vi "一体站流程自动启动.vi"(11 "参数":T1={"CODCr"={"启动测量模式"={"测量模式"=enum."水样测量"}, "确定按钮"=TRUE}, "参数启用"={"多参数"=FALSE, "CODMn"=FALSE, "总磷总氮"=FALSE, "氨氮"=FALSE, "CODcr"=FALSE}}) -> ()   [LabVIEW 2016, in "PLC.lvlib"]
uses:
  PLC.lvlib
  API/CodCr/CodCr.lvlib
panel:
  out "枚举":enum16{"初始化", "采配水启动", "等待", "配水", "排水", "结束"}(ring)
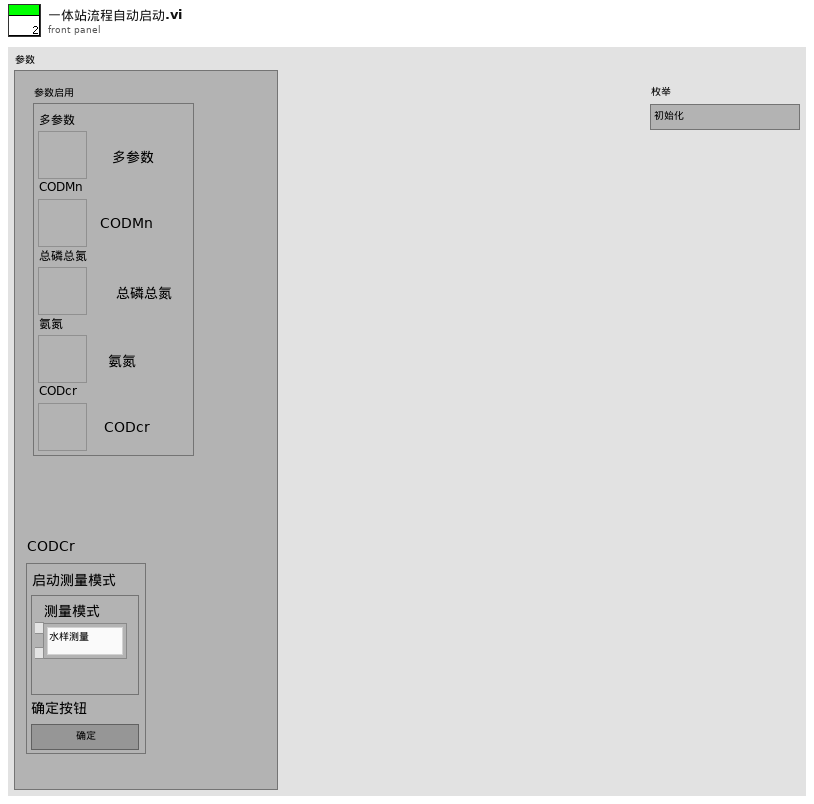
[diagram p1: front panel]
types:
  T1 = cluster{"CODCr":cluster{"启动测量模式":cluster{"测量模式":enum16{"水样测量", "标样核查", "零点核查", "加标回收", "平行样", "校零", "校标"}}, "确定按钮":bool}, "参数启用":cluster{"多参数":bool, "CODMn":bool, "总磷总氮":bool, "氨氮":bool, "CODcr":bool}}
  T2 = cluster{"命令":string, cluster{"starting address":u16, "holding register value":u16}}
  T3 = enum16{"待机", "启动氨氮", "氨氮测量中", "启动总磷", "总磷测量中", "结束"}
  T4 = cluster{"站号":u16, "量程切换":enum32{"H", "L", "AUTO"}, "控制命令":enum16{"启动测量", "标样核查", "零点核查", "跨度核查", "空白测试", "平行样测试", "加标回收", "空白校准", "标样校准", "初始化（清洗）", "停止测试", "仪器重启", "校时", "模式设置", "测量间隔设置"}, "模式设置":enum16{"待机", "连续模式", "周期模式", "定点模式", "受控模式", "手动模式"}, "测量间隔":u16}
  T5 = cluster{"时间标识":timestamp, "设备":string, "日志信息":string}
  T6 = cluster{"站号":u16, "量程切换":enum32{"H", "L", "AUTO"}, "控制命令":enum16{"启动测量", "标样核查", "零点核查", "跨度核查", "空白测试", "平行样测试", "加标回收", "空白校准", "标样校准", "初始化（清洗）", "停止测试", "仪器重启", "校时", "模式设置", "测量间隔设置", "盲样测试"}, "模式设置":enum16{"待机", "连续模式", "周期模式", "定点模式", "受控模式", "手动模式"}, "测量间隔":u16}
  T7 = enum16{"空闲", "水样测试", "标样核查", "零点核查", "跨度核查", "空白测试", "平行样测试", "加标回收", "空白校准", "标样校准", "初始化（清洗）"}
  T8 = cluster{"测量模式":enum16{"待机", "水样测试", "标样核查", "零点核查", "跨度核查", "空白测试", "平行样测试", "加标回收", "空白校准", "标样校准", "初始化（清洗）"}, "数据标记表":string, "测量时间":dbl}
  T9 = enum16{"待机", "水样测试", "标样核查", "零点核查", "跨度核查", "空白测试", "平行样测试", "加标回收", "空白校准", "标样校准", "初始化（清洗）"}
  T10 = cluster{"R0":i16, "R1":i16, "R2":i16, "R3":i16, "R4":i16, "R5":i16, "R6":i16, "R7":i16, "R8":i16, "R9":i16, "R10":i16, "R11":i16, "R12":i16, "R13":i16, "R14":i16, "R15":i16, "R16":i16, "R17":i16, "R18":i16, "R19":i16, "R20":i16, "R21":i16, "R22":i16}
  T11 = enum32{"Bad", "Idle", "Run top level", "Running"}
  T12 = cluster{"测量模式":enum16{"水样测量", "标样核查", "零点核查", "加标回收", "平行样", "校零", "校标"}}
  T13 = cluster{"系统时间":timestamp, "工作状态":enum16{"空闲", "水样测试", "标样核查", "零点核查", "跨度核查", "空白测试", "平行样测试", "加标回收", "空白校准", "标样校准", "初始化（清洗）"}, "测量模式":enum16{"待机", "连续模式", "周期模式", "定点模式", "受控模式", "手动模式"}, "告警代码":enum16{"无告警", "缺试剂告警", "缺水样告警", "缺蒸馏水告警", "缺标液告警", "仪表漏液告警", "标定异常告警", "超量程告警", "加热异常", "低试剂预警", "超上限告警", "超下限告警", "仪表内部其他异常", "滴定异常告警", "电极异常告警", "量程切换告警", "参数设置告警", "PH电极电位异常", "电导率电极异常", "浊度光度异常", "溶解氧电极异常", "溶解氧光强异常", "温度异常告警", "PH异常告警", "溶解氧异常告警", "电导率异常告警", "浊度异常告警", "叶绿素异常告警", "藻密度异常告警", "蓝绿藻异常告警", "ORP异常告警", "氨氮异常告警", "清洁刷异常告警", "SD卡异常告警", "蓝牙异常告警", "Wifi异常告警", "流程异常告警"}, "故障代码":enum16{"无故障", "电机故障", "温度故障", "通讯故障", "滴定故障"}, "日志代码":u16, "软件版本":u16, "F0":sgl, "F1":sgl, "F2":sgl, "F3":sgl, "T":sgl, "H":sgl, "id":u16, "flowid":u16, "量程":u16}
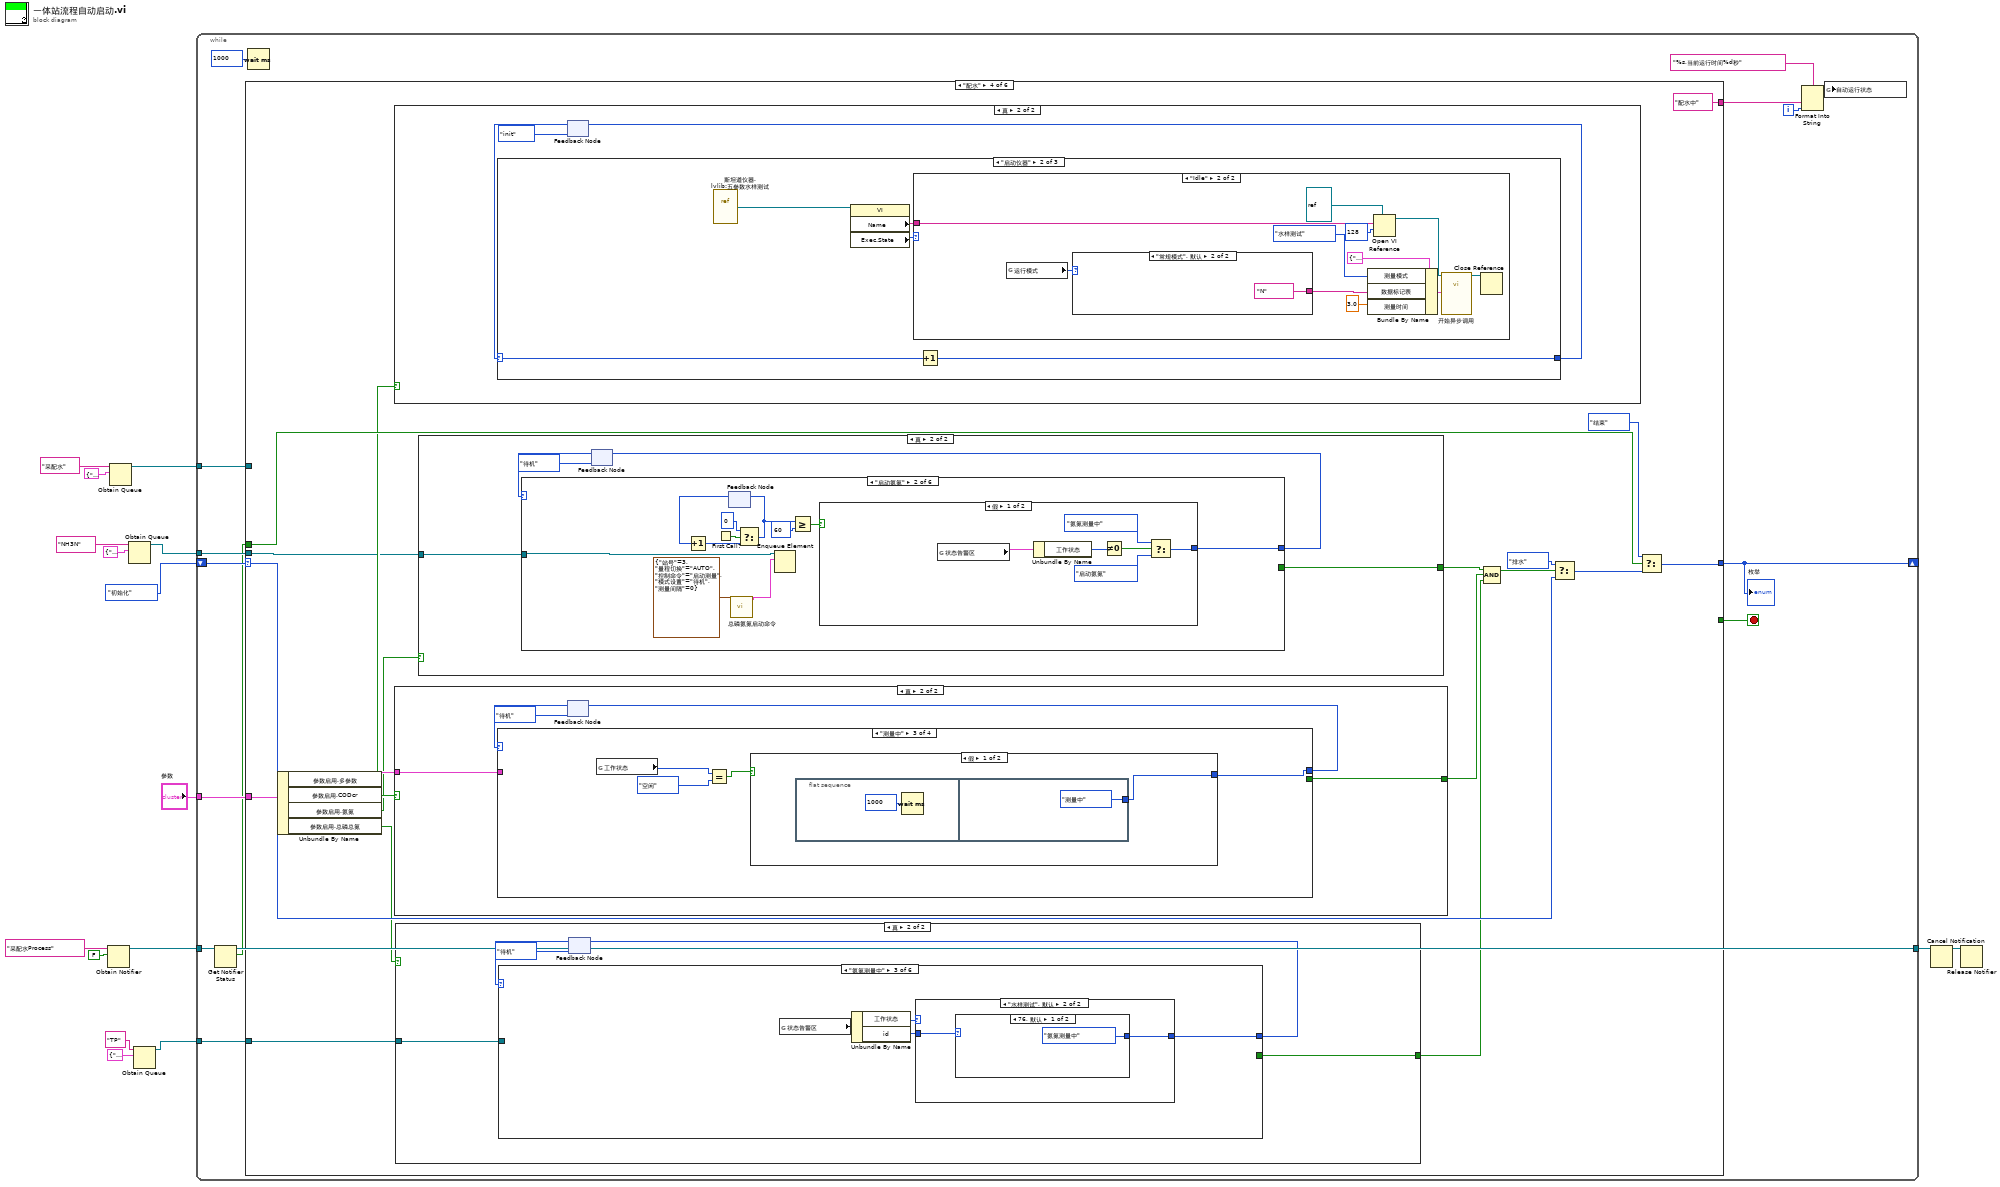
[diagram p0: block diagram]
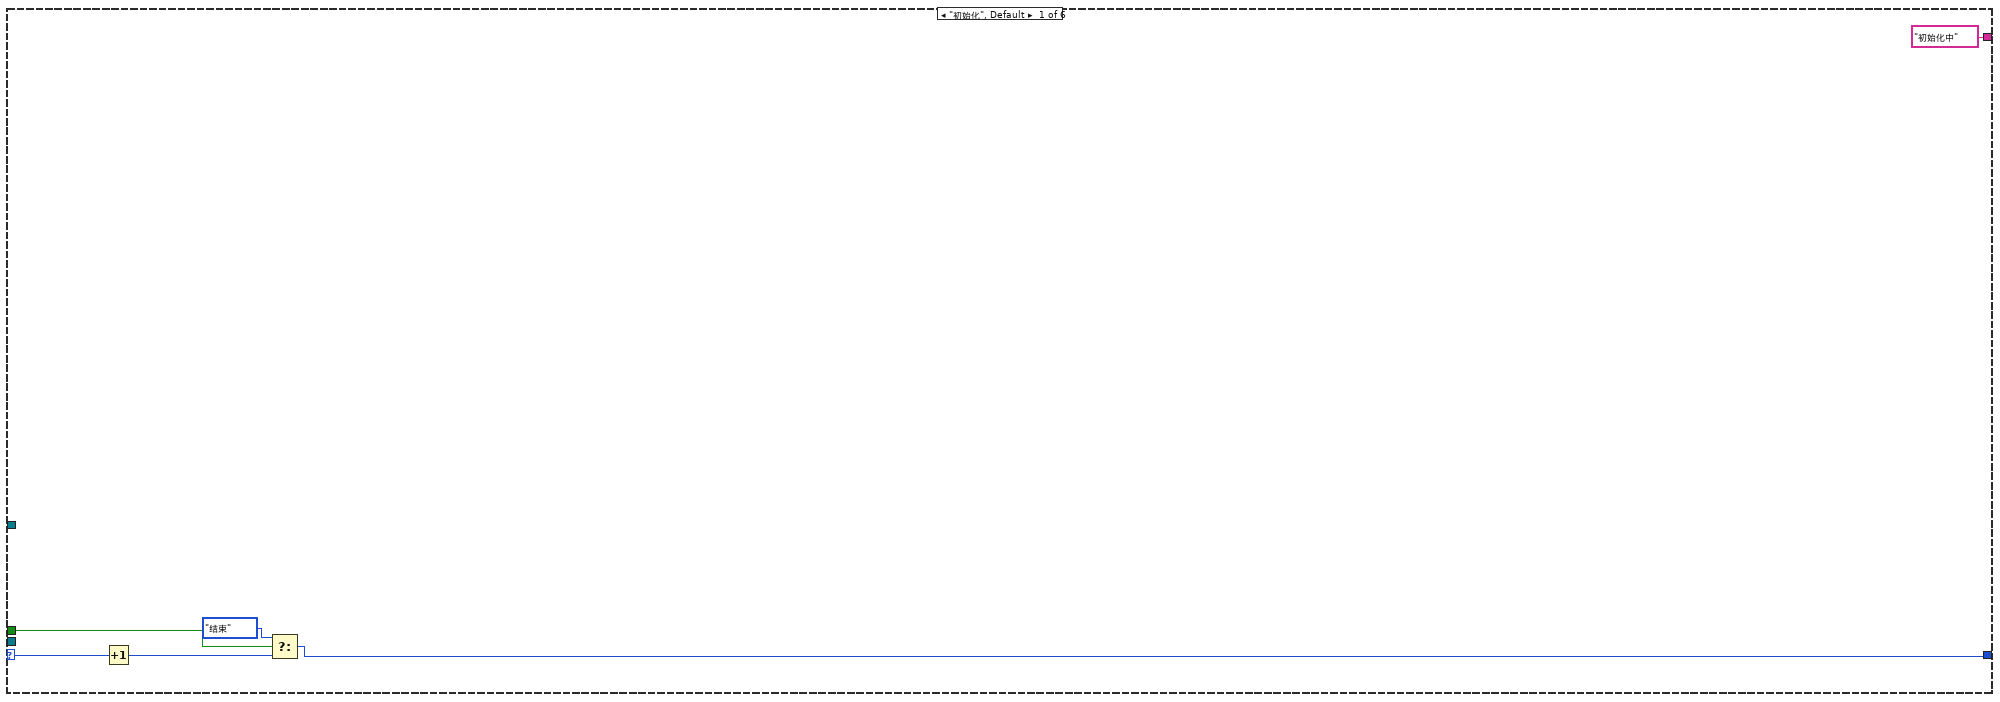
[diagram p2: hidden frame]
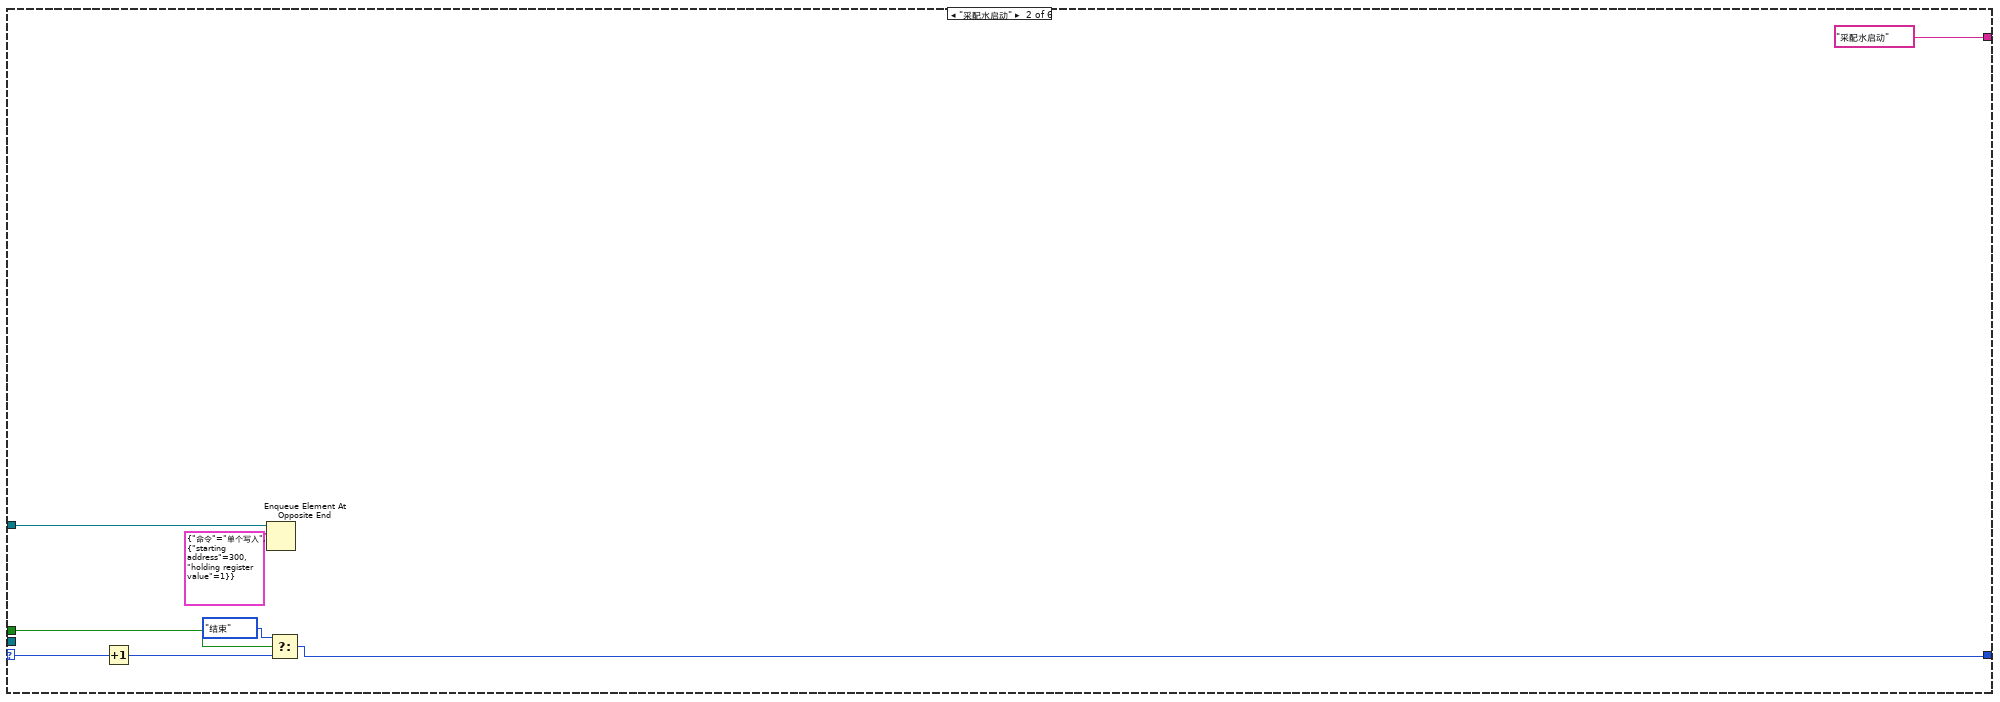
[diagram p3: hidden frame]
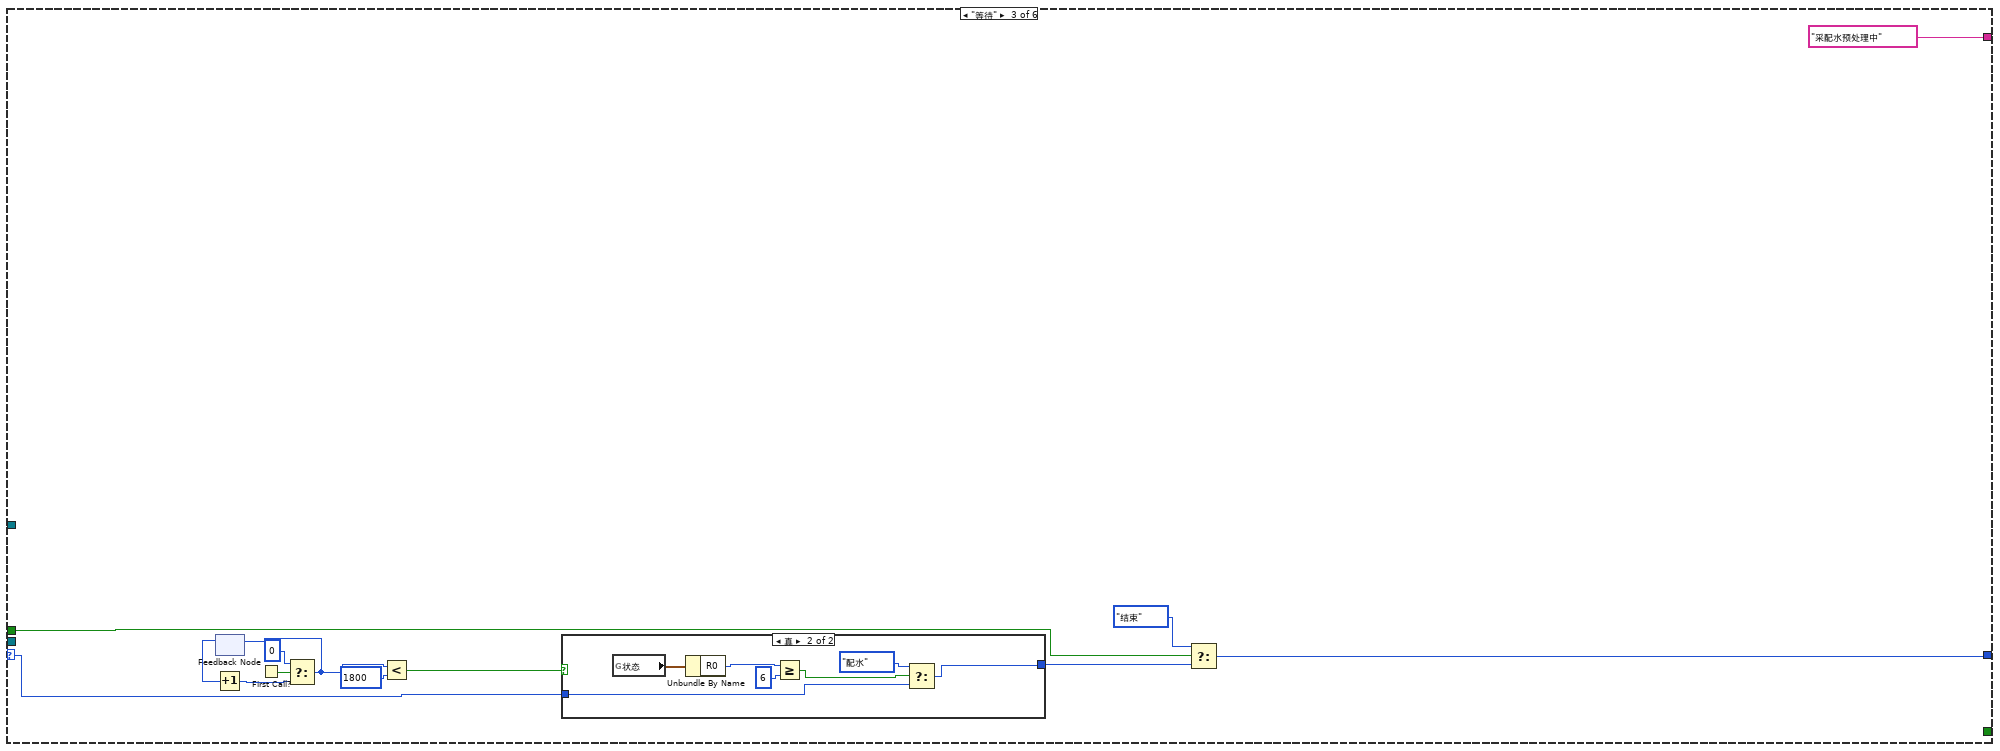
[diagram p4: hidden frame]
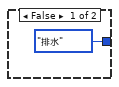
[diagram p5: hidden frame]
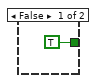
[diagram p6: hidden frame]
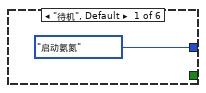
[diagram p7: hidden frame]
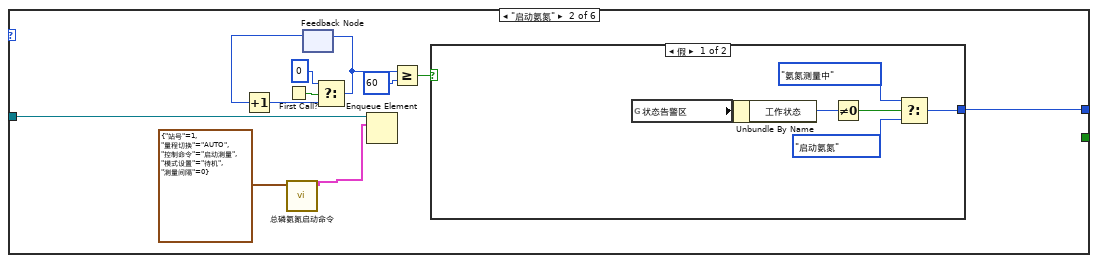
[diagram p8: hidden frame]
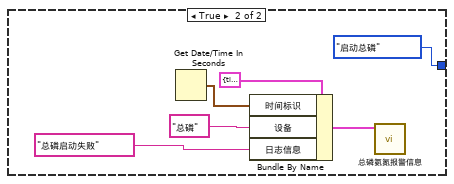
[diagram p9: hidden frame]
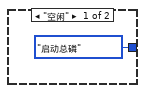
[diagram p10: hidden frame]
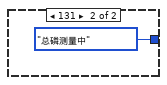
[diagram p11: hidden frame]
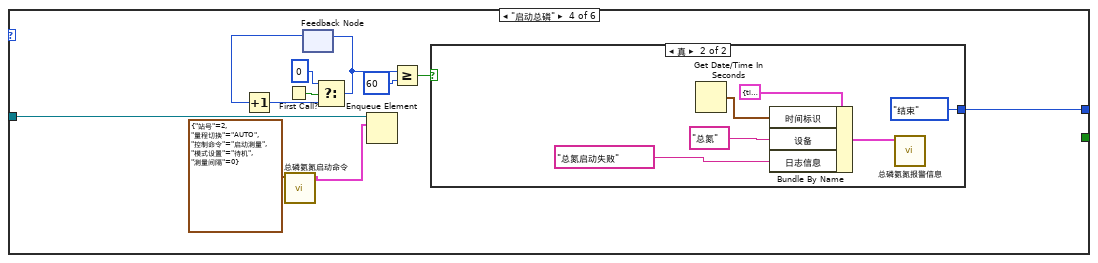
[diagram p12: hidden frame]
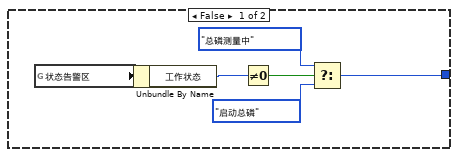
[diagram p13: hidden frame]
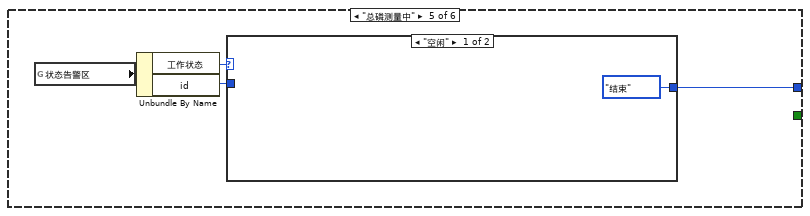
[diagram p14: hidden frame]
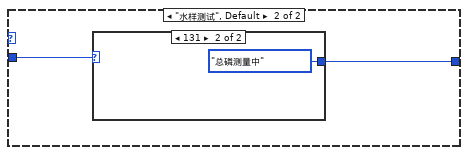
[diagram p15: hidden frame]
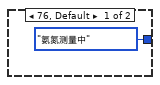
[diagram p16: hidden frame]
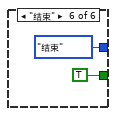
[diagram p17: hidden frame]
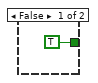
[diagram p18: hidden frame]
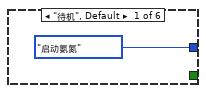
[diagram p19: hidden frame]
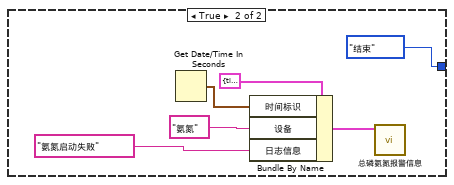
[diagram p20: hidden frame]
diagram:
  n1 = Obtain Notifier(name (unnamed)="采配水Process" ("名称（未命名）"), notification data type=FALSE) -> (notifier out=w7:refnum<notifier>)  [unwired: 2 in, 2 out]
  n2 = Obtain Queue(name (unnamed)="采配水" ("名称（未命名）"), element data type=cluster{"命令":string, "数据":variant} {"命令"="", "数据"=variant}) -> (queue out=w14:refnum<queue>)  [unwired: 3 in, 2 out]
  n3 = Obtain Queue(name (unnamed)="NH3N" ("名称（未命名）"), element data type=cluster{"命令":string, "data":variant} {"命令"="", "data"=variant}) -> (queue out=w2:refnum<queue>)  [unwired: 3 in, 2 out]
  n4 = Obtain Queue(name (unnamed)="TP" ("名称（未命名）"), element data type=cluster{"命令":string, "data":variant} {"命令"="", "data"=variant}) -> (queue out=w1:refnum<queue>)  [unwired: 3 in, 2 out]
  n5 = while {
    tunnel: w14 -> [w31]
    shift-right: [w29] -> _
    shift-left: enum16{"初始化", "采配水启动", "等待", "配水", "排水", "结束"}."初始化" ("枚举") -> [w30]
    tunnel: w2 -> [w27]
    tunnel: "参数" -> [w26]
    tunnel: w7 -> [w25]
    tunnel: [w24] -> w6
    tunnel: w1 -> [w17]
    i -> [w21]
    stop <- w19 stop-if-true
    n6 = Get Notifier Status(notifier=w25) -> (notifier out=w24:refnum<notifier>, current notification=w18:bool)  [unwired: 1 in, 3 out]
    n7 = case shown="\"配水\"" w30 {
      selector: w30 -> [w37 w43 w56 w83 w286 w292]
      tunnel: w31 -> [_ w44 _ _ w287 _]
      tunnel: [w33 w38 w46 w77 w281 w291] -> w29
      tunnel: [_ _ _ _ _ TRUE] -> w19
      tunnel: w27 -> [_ _ _ w71 _ _]
      tunnel: w26 -> [_ _ _ w82 _ _]
      tunnel: ["初始化中" ("输入 1") "采配水启动" ("输入 1") "采配水预处理中" ("输入 1") "配水中" ("输入 1") "排水中" ("输入 1") "结束" ("输入 1")] -> w22
      tunnel: w18 -> [w35 w40 w48 w79 w283 _]
      tunnel: w17 -> [_ _ _ w72 _ _]
      frame "初始化", Default {
        n8 = Increment(x=w37) -> (x+1=w34:enum16{"初始化", "采配水启动", "等待", "配水", "排水", "结束"})
        n9 = Select(t=enum16{"初始化", "采配水启动", "等待", "配水", "排水", "结束"}."结束", s=w35, f=w34) -> (s? t:f=w33:enum16{"初始化", "采配水启动", "等待", "配水", "排水", "结束"})
      }
      frame "采配水启动" {
        n10 = Increment(x=w43) -> (x+1=w39:enum16{"初始化", "采配水启动", "等待", "配水", "排水", "结束"})
        n11 = Enqueue Element At Opposite End(queue=w44, element=T2 {"命令"="单个写入", {"starting address"=300, "holding register value"=1}} ("元素")) -> ()  [unwired: 2 in, 3 out]
        n12 = Select(t=enum16{"初始化", "采配水启动", "等待", "配水", "排水", "结束"}."结束", s=w40, f=w39) -> (s? t:f=w38:enum16{"初始化", "采配水启动", "等待", "配水", "排水", "结束"})
      }
      frame "等待" {
        n13 = feedback #1() -> (w53:i32)  [unwired: 1 in]
        n14 = Increment(x=w53) -> (x+1=w52:i32)
        n15 = First Call?() -> (First Call?: T/F=w54:bool)
        n16 = Select(t=0, s=w54, f=w52) -> (s? t:f=w51:i32)
        n17 = feedback-in #1(w51) -> ()
        n18 = Less?(x=w51, y=1800) -> (x < y?=w57:bool)
        n19 = case shown="真" w57 {
          tunnel: w56 -> [_ w61]
          tunnel: [enum16{"初始化", "采配水启动", "等待", "配水", "排水", "结束"}."排水" ("枚举") w60] -> w47
          frame False {
          }
          frame True {
            n20 = global read "采配水全局变量.vi" "状态"() -> (w66:T10)
            n21 = Unbundle By Name(w66) -> ("R0"=w65:i16)
            n22 = Greater Or Equal?(x=w65, y=i16 6) -> (x >= y?=w63:bool)
            n23 = Select(t=enum16{"初始化", "采配水启动", "等待", "配水", "排水", "结束"}."配水" ("枚举"), s=w63, f=w61) -> (s? t:f=w60:enum16{"初始化", "采配水启动", "等待", "配水", "排水", "结束"})
          }
        }
        n24 = Select(t=enum16{"初始化", "采配水启动", "等待", "配水", "排水", "结束"}."结束", s=w48, f=w47) -> (s? t:f=w46:enum16{"初始化", "采配水启动", "等待", "配水", "排水", "结束"})
      }
      frame "配水" {
        n25 = Unbundle By Name(w82) -> ("参数启用.多参数"=w76:bool, "参数启用.CODcr"=w75:bool, "参数启用.氨氮"=w74:bool, "参数启用.总磷总氮"=w73:bool)
        n26 = case shown="真" w76 {
          frame False {
          }
          frame True {
            n27 = feedback #2(enum16{"init", "启动仪器", "测量中"}."init") -> (w258:enum16{"init", "启动仪器", "测量中"})
            n28 = case shown="\"启动仪器\"" w258 {
              selector: w258 -> [w261 w266 _]
              tunnel: [w260 w265 enum16{"init", "启动仪器", "测量中"}."测量中"] -> w259
              frame "init", Default {
                n29 = Increment(x=w261) -> (x+1=w260:enum16{"init", "启动仪器", "测量中"})
              }
              frame "启动仪器" {
                n30 = vi-ref "斯坦道仪器.lvlib:五参数水样测试.vi"() -> (w263:refnum<vi>)
                n31 = property class="VI"(reference=w263) -> ("Name"=w262:string, "Exec.State"=w264:T11)  [unwired: 1 in, 2 out]
                n32 = case shown="\"Idle\"" w264 {
                  tunnel: w262 -> [_ w273]
                  frame "Bad", Default {
                  }
                  frame "Idle" {
                    n33 = global read "系统变量.vi" "运行模式"() -> (w268:enum16{"维护模式", "常规模式", "应急模式", "质控模式"})
                    n34 = case shown="\"常规模式\", 默认" w268 {
                      tunnel: ["M" ("数据标记表") "N" ("数据标记表")] -> w267
                      frame "维护模式" {
                      }
                      frame "常规模式", Default {
                      }
                    }
                    n35 = Bundle By Name(cluster=T8 {"测量模式"=enum."待机", "数据标记表"="", "测量时间"=0.0} ("启动参数"), "测量模式"=T9."水样测试", "数据标记表"=w267, "测量时间"=3.0) -> (w269:T8)
                    n36 = Open VI Reference(type specifier VI Refnum (for type only)=refnum<vi> refnum ("类型说明符VI引用句柄（仅用于类型）"), vi path=w273, options=128 ("选项")) -> (vi reference=w272:refnum<vi>)  [unwired: 3 in, 1 out]
                    n37 = call-by-ref "开始异步调用"(reference=w272, "启动参数"=w269) -> (reference out=w271:refnum<vi>)  [unwired: 12 in, 1 out]
                    n38 = Close Reference(reference=w271) -> ()  [unwired: 1 in, 1 out]
                  }
                }
                n39 = Increment(x=w266) -> (x+1=w265:enum16{"init", "启动仪器", "测量中"})
              }
              frame "测量中" {
              }
            }
            n40 = feedback-in #2(w259) -> ()
          }
        }
        n41 = case shown="真" w75 {
          tunnel: [TRUE w233] -> w69
          tunnel: w82 -> [_ w232]
          frame False {
          }
          frame True {
            n42 = feedback #3(enum16{"待机", "启动测量", "测量中", "结束"}."待机") -> (w235:enum16{"待机", "启动测量", "测量中", "结束"})
            n43 = case shown="\"测量中\"" w235 {
              tunnel: [enum16{"待机", "启动测量", "测量中", "结束"}."启动测量" w241 w250 enum16{"待机", "启动测量", "测量中", "结束"}."结束"] -> w234
              tunnel: w232 -> [_ w242 _ _]
              tunnel: [_ _ _ TRUE] -> w233
              frame "待机", Default {
              }
              frame "启动测量" {
                n44 = Unbundle By Name(w242) -> ("CODCr.启动测量模式"=w240:T12)
                n45 = global read "CODCr工作状态.vi" "工作状态"() -> (w239:T7)
                n46 = call "CODCr启动命令 (子VI).vi"("启动测量模式"=w240) -> ()  [unwired: 11 in]
                n47 = Not Equal To 0?(x=w239) -> (x != 0?=w238:bool)
                n48 = case shown="假" w238 {
                  tunnel: [w243 enum16{"待机", "启动测量", "测量中", "结束"}."测量中"] -> w241
                  frame False {
                    n49 = flat-sequence {
                      tunnel: [enum16{"待机", "启动测量", "测量中", "结束"}."启动测量"] -> w243
                      frame #0 {
                        n50 = Wait (ms)(milliseconds to wait=u32 1000 ("等待时间（毫秒）")) -> ()  [unwired: 1 out]
                      }
                      frame #1 {
                      }
                    }
                  }
                  frame True {
                  }
                }
              }
              frame "测量中" {
                n51 = global read "CODCr工作状态.vi" "工作状态"() -> (w249:T7)
                n52 = Equal?(x=w249, y=T7."空闲" ("工作状态")) -> (x = y?=w248:bool)
                n53 = case shown="假" w248 {
                  tunnel: [w251 enum16{"待机", "启动测量", "测量中", "结束"}."结束"] -> w250
                  frame False {
                    n54 = flat-sequence {
                      tunnel: [enum16{"待机", "启动测量", "测量中", "结束"}."测量中"] -> w251
                      frame #0 {
                        n55 = Wait (ms)(milliseconds to wait=u32 1000 ("等待时间（毫秒）")) -> ()  [unwired: 1 out]
                      }
                      frame #1 {
                      }
                    }
                  }
                  frame True {
                  }
                }
              }
              frame "结束" {
              }
            }
            n56 = feedback-in #3(w234) -> ()
          }
        }
        n57 = case shown="真" w73 {
          tunnel: w72 -> [_ w87]
          tunnel: [TRUE w86] -> w67
          frame False {
          }
          frame True {
            n58 = feedback #4(T3."待机") -> (w89:T3)
            n59 = case shown="\"氨氮测量中\"" w89 {
              tunnel: [T3."启动氨氮" w101 w115 w133 w147 T3."结束"] -> w88
              tunnel: w87 -> [_ w102 _ w134 _ _]
              tunnel: [_ _ _ _ _ TRUE] -> w86
              frame "待机", Default {
              }
              frame "启动氨氮" {
                n60 = First Call?() -> (First Call?: T/F=w99:bool)
                n61 = call "总磷氨氮启动命令.vi"("参数"=T4 {"站号"=1, "量程切换"=enum."AUTO", "控制命令"=enum."启动测量", "模式设置"=enum."待机", "测量间隔"=0}) -> ("启动命令"=w92:cluster{"命令":string, "data":variant})  [unwired: 10 in]
                n62 = feedback #5() -> (w98:i32)  [unwired: 1 in]
                n63 = Increment(x=w98) -> (x+1=w97:i32)
                n64 = Select(t=0, s=w99, f=w97) -> (s? t:f=w96:i32)
                n65 = feedback-in #5(w96) -> ()
                n66 = Enqueue Element(queue=w102, element=w92) -> ()  [unwired: 2 in, 3 out]
                n67 = Greater Or Equal?(x=w96, y=60) -> (x >= y?=w94:bool)
                n68 = case shown="假" w94 {
                  tunnel: [w105 T3."启动总磷"] -> w101
                  frame False {
                    n69 = global read "VAR总磷氨氮全局变量.vi" "状态告警区"() -> (w108:T13)
                    n70 = Unbundle By Name(w108) -> ("工作状态"=w107:T7)
                    n71 = Not Equal To 0?(x=w107) -> (x != 0?=w106:bool)
                    n72 = Select(t=T3."氨氮测量中", s=w106, f=T3."启动氨氮") -> (s? t:f=w105:T3)
                  }
                  frame True {
                    n73 = Get Date/Time In Seconds() -> (seconds since 1Jan1904=w113:timestamp)
                    n74 = Bundle By Name(cluster=T5 {"时间标识"=timestamp(0 s since 1904-01-01), "设备"="", "日志信息"=""} ("data in"), "时间标识"=w113, "设备"="总磷", "日志信息"="总磷启动失败") -> (w109:T5)
                    n75 = call "总磷氨氮报警信息.vi"("data in"=w109) -> ()  [unwired: 11 in]
                  }
                }
              }
              frame "氨氮测量中" {
                n76 = global read "VAR总磷氨氮全局变量.vi" "状态告警区"() -> (w118:T13)
                n77 = Unbundle By Name(w118) -> ("工作状态"=w117:T7, "id"=w116:u16)
                n78 = case shown="\"水样测试\", 默认" w117 {
                  tunnel: [T3."启动总磷" w120] -> w115
                  tunnel: w116 -> [_ w121]
                  frame "空闲" {
                  }
                  frame "水样测试", Default {
                    n79 = case shown="76, 默认" w121 {
                      tunnel: [T3."氨氮测量中" T3."总磷测量中"] -> w120
                      frame 76, Default {
                      }
                      frame 131 {
                      }
                    }
                  }
                }
              }
              frame "启动总磷" {
                n80 = First Call?() -> (First Call?: T/F=w131:bool)
                n81 = call "总磷氨氮启动命令.vi"("参数"=T4 {"站号"=2, "量程切换"=enum."AUTO", "控制命令"=enum."启动测量", "模式设置"=enum."待机", "测量间隔"=0}) -> ("启动命令"=w124:cluster{"命令":string, "data":variant})  [unwired: 10 in]
                n82 = feedback #6() -> (w130:i32)  [unwired: 1 in]
                n83 = Increment(x=w130) -> (x+1=w129:i32)
                n84 = Select(t=0, s=w131, f=w129) -> (s? t:f=w128:i32)
                n85 = feedback-in #6(w128) -> ()
                n86 = Enqueue Element(queue=w134, element=w124) -> ()  [unwired: 2 in, 3 out]
                n87 = Greater Or Equal?(x=w128, y=60) -> (x >= y?=w126:bool)
                n88 = case shown="真" w126 {
                  tunnel: [w137 T3."结束"] -> w133
                  frame False {
                    n89 = global read "VAR总磷氨氮全局变量.vi" "状态告警区"() -> (w138:T13)
                    n90 = Unbundle By Name(w138) -> ("工作状态"=w139:T7)
                    n91 = Not Equal To 0?(x=w139) -> (x != 0?=w140:bool)
                    n92 = Select(t=T3."总磷测量中", s=w140, f=T3."启动总磷") -> (s? t:f=w137:T3)
                  }
                  frame True {
                    n93 = Get Date/Time In Seconds() -> (seconds since 1Jan1904=w146:timestamp)
                    n94 = Bundle By Name(cluster=T5 {"时间标识"=timestamp(0 s since 1904-01-01), "设备"="", "日志信息"=""} ("data in"), "时间标识"=w146, "设备"="总氮", "日志信息"="总氮启动失败") -> (w141:T5)
                    n95 = call "总磷氨氮报警信息.vi"("data in"=w141) -> ()  [unwired: 11 in]
                  }
                }
              }
              frame "总磷测量中" {
                n96 = global read "VAR总磷氨氮全局变量.vi" "状态告警区"() -> (w150:T13)
                n97 = Unbundle By Name(w150) -> ("工作状态"=w149:T7, "id"=w148:u16)
                n98 = case shown="\"空闲\"" w149 {
                  tunnel: [T3."结束" w152] -> w147
                  tunnel: w148 -> [_ w153]
                  frame "空闲" {
                  }
                  frame "水样测试", Default {
                    n99 = case shown="131" w153 {
                      tunnel: [T3."氨氮测量中" T3."总磷测量中"] -> w152
                      frame 76, Default {
                      }
                      frame 131 {
                      }
                    }
                  }
                }
              }
              frame "结束" {
              }
            }
            n100 = feedback-in #4(w88) -> ()
          }
        }
        n101 = case shown="真" w74 {
          tunnel: [TRUE w160] -> w70
          tunnel: w71 -> [_ w159]
          frame False {
          }
          frame True {
            n102 = feedback #7(T3."待机") -> (w162:T3)
            n103 = case shown="\"启动氨氮\"" w162 {
              tunnel: [T3."启动氨氮" w175 w189 w207 w221 T3."结束"] -> w161
              tunnel: [_ _ _ _ _ TRUE] -> w160
              tunnel: w159 -> [_ w165 _ w197 _ _]
              frame "待机", Default {
              }
              frame "启动氨氮" {
                n104 = First Call?() -> (First Call?: T/F=w173:bool)
                n105 = feedback #8() -> (w172:i32)  [unwired: 1 in]
                n106 = Increment(x=w172) -> (x+1=w171:i32)
                n107 = call "总磷氨氮启动命令.vi"("参数"=T6 {"站号"=3, "量程切换"=enum."AUTO", "控制命令"=enum."启动测量", "模式设置"=enum."待机", "测量间隔"=0}) -> ("启动命令"=w166:cluster{"命令":string, "data":variant})  [unwired: 10 in]
                n108 = Select(t=0, s=w173, f=w171) -> (s? t:f=w170:i32)
                n109 = feedback-in #8(w170) -> ()
                n110 = Enqueue Element(queue=w165, element=w166) -> ()  [unwired: 2 in, 3 out]
                n111 = Greater Or Equal?(x=w170, y=60) -> (x >= y?=w168:bool)
                n112 = case shown="假" w168 {
                  tunnel: [w179 T3."结束"] -> w175
                  frame False {
                    n113 = global read "VAR总磷氨氮全局变量.vi" "状态告警区"() -> (w176:T13)
                    n114 = Unbundle By Name(w176) -> ("工作状态"=w181:T7)
                    n115 = Not Equal To 0?(x=w181) -> (x != 0?=w180:bool)
                    n116 = Select(t=T3."氨氮测量中", s=w180, f=T3."启动氨氮") -> (s? t:f=w179:T3)
                  }
                  frame True {
                    n117 = Get Date/Time In Seconds() -> (seconds since 1Jan1904=w186:timestamp)
                    n118 = Bundle By Name(cluster=T5 {"时间标识"=timestamp(0 s since 1904-01-01), "设备"="", "日志信息"=""} ("data in"), "时间标识"=w186, "设备"="氨氮", "日志信息"="氨氮启动失败") -> (w182:T5)
                    n119 = call "总磷氨氮报警信息.vi"("data in"=w182) -> ()  [unwired: 11 in]
                  }
                }
              }
              frame "氨氮测量中" {
                n120 = global read "VAR总磷氨氮全局变量.vi" "状态告警区"() -> (w188:T13)
                n121 = Unbundle By Name(w188) -> ("工作状态"=w191:T7, "id"=w190:u16)
                n122 = case shown="\"水样测试\", 默认" w191 {
                  tunnel: [T3."结束" w193] -> w189
                  tunnel: w190 -> [_ w194]
                  frame "空闲" {
                  }
                  frame "水样测试", Default {
                    n123 = case shown="76, 默认" w194 {
                      tunnel: [T3."氨氮测量中" T3."总磷测量中"] -> w193
                      frame 76, Default {
                      }
                      frame 131 {
                      }
                    }
                  }
                }
              }
              frame "启动总磷" {
                n124 = First Call?() -> (First Call?: T/F=w205:bool)
                n125 = feedback #9() -> (w204:i32)  [unwired: 1 in]
                n126 = Increment(x=w204) -> (x+1=w203:i32)
                n127 = call "总磷氨氮启动命令.vi"("参数"=T6 {"站号"=1, "量程切换"=enum."AUTO", "控制命令"=enum."启动测量", "模式设置"=enum."待机", "测量间隔"=0}) -> ("启动命令"=w199:cluster{"命令":string, "data":variant})  [unwired: 10 in]
                n128 = Select(t=0, s=w205, f=w203) -> (s? t:f=w202:i32)
                n129 = feedback-in #9(w202) -> ()
                n130 = Enqueue Element(queue=w197, element=w199) -> ()  [unwired: 2 in, 3 out]
                n131 = Greater Or Equal?(x=w202, y=60) -> (x >= y?=w200:bool)
                n132 = case shown="假" w200 {
                  tunnel: [w211 T3."结束"] -> w207
                  frame False {
                    n133 = global read "VAR总磷氨氮全局变量.vi" "状态告警区"() -> (w208:T13)
                    n134 = Unbundle By Name(w208) -> ("工作状态"=w212:T7)
                    n135 = Not Equal To 0?(x=w212) -> (x != 0?=w213:bool)
                    n136 = Select(t=T3."总磷测量中", s=w213, f=T3."启动总磷") -> (s? t:f=w211:T3)
                  }
                  frame True {
                    n137 = Get Date/Time In Seconds() -> (seconds since 1Jan1904=w219:timestamp)
                    n138 = Bundle By Name(cluster=T5 {"时间标识"=timestamp(0 s since 1904-01-01), "设备"="", "日志信息"=""} ("data in"), "时间标识"=w219, "设备"="总磷", "日志信息"="总磷启动失败") -> (w214:T5)
                    n139 = call "总磷氨氮报警信息.vi"("data in"=w214) -> ()  [unwired: 11 in]
                  }
                }
              }
              frame "总磷测量中" {
                n140 = global read "VAR总磷氨氮全局变量.vi" "状态告警区"() -> (w220:T13)
                n141 = Unbundle By Name(w220) -> ("工作状态"=w223:T7, "id"=w222:u16)
                n142 = case shown="\"水样测试\", 默认" w223 {
                  tunnel: [T3."结束" w225] -> w221
                  tunnel: w222 -> [_ w226]
                  frame "空闲" {
                  }
                  frame "水样测试", Default {
                    n143 = case shown="76, 默认" w226 {
                      tunnel: [T3."氨氮测量中" T3."总磷测量中"] -> w225
                      frame 76, Default {
                      }
                      frame 131 {
                      }
                    }
                  }
                }
              }
              frame "结束" {
              }
            }
            n144 = feedback-in #7(w161) -> ()
          }
        }
        n145 = Compound Arithmetic op=AND ("复合运算")(w70, w69, w67) -> (w68:bool)
        n146 = Select(t=enum16{"初始化", "采配水启动", "等待", "配水", "排水", "结束"}."排水" ("枚举"), s=w68, f=w83) -> (s? t:f=w78:enum16{"初始化", "采配水启动", "等待", "配水", "排水", "结束"})
        n147 = Select(t=enum16{"初始化", "采配水启动", "等待", "配水", "排水", "结束"}."结束", s=w79, f=w78) -> (s? t:f=w77:enum16{"初始化", "采配水启动", "等待", "配水", "排水", "结束"})
      }
      frame "排水" {
        n148 = Increment(x=w286) -> (x+1=w282:enum16{"初始化", "采配水启动", "等待", "配水", "排水", "结束"})
        n149 = Enqueue Element At Opposite End(queue=w287, element=T2 {"命令"="单个写入", {"starting address"=303, "holding register value"=1}} ("元素")) -> ()  [unwired: 2 in, 3 out]
        n150 = Select(t=enum16{"初始化", "采配水启动", "等待", "配水", "排水", "结束"}."结束", s=w283, f=w282) -> (s? t:f=w281:enum16{"初始化", "采配水启动", "等待", "配水", "排水", "结束"})
      }
      frame "结束" {
        n151 = Increment(x=w292) -> (x+1=w291:enum16{"初始化", "采配水启动", "等待", "配水", "排水", "结束"})
      }
    }
    "枚举" <- w29
    n152 = Wait (ms)(milliseconds to wait=u32 1000 ("等待时间（毫秒）")) -> ()  [unwired: 1 out]
    n153 = Format Into String(format string="%s,当前运行时间%d秒" ("格式字符串"), w22, w21) -> (resulting string=w20:string)  [unwired: 2 in, 1 out]
    n154 = global write "采配水全局变量.vi" "自动运行状态"(w20) -> ()
  }
  n155 = Cancel Notification(0:w6) -> (8:w5:refnum<notifier>)  [unwired: 1 in, 2 out]
  n156 = Release Notifier(notifier=w5) -> ()  [unwired: 2 in, 3 out]
